vi "Close Network Interface.vi"(8 "error in (no error)":errorcluster, 11 "Network Interface":refnum<data-value>) -> (0 "error out":errorcluster)   [LabVIEW 2017, in "Network Interface.lvlib" / "Network Interface.lvclass"]
uses:
  <vilib>/gpm_packages/@cs/Network-Sink/Source/Network Interface/Network Interface/Network Interface.lvclass
  <vilib>/gpm_packages/@cs/Network-Sink/Source/Network Interface/Network Session Handler/Session Handler Message Names ENUM.ctl
  <vilib>/gpm_packages/@cs/Network-Sink/Source/Network Interface/Network Interface/Network Interface.lvclass/Network Interface.ctl
  <vilib>/gpm_packages/@cs/Network-Sink/Source/Network Interface/Message Queue/Message Queue.lvclass/Message Queue.ctl
  05c7863f-13bf-43fd-8f9a-3362d466c09a.vi
  <vilib>/gpm_packages/@cs/Network-Sink/Source/Network Interface/Message Queue/Protected Enqueue.vi
  <vilib>/gpm_packages/@cs/Network-Sink/Source/Network Interface/Network Session Handler/Network Session Handler.lvclass
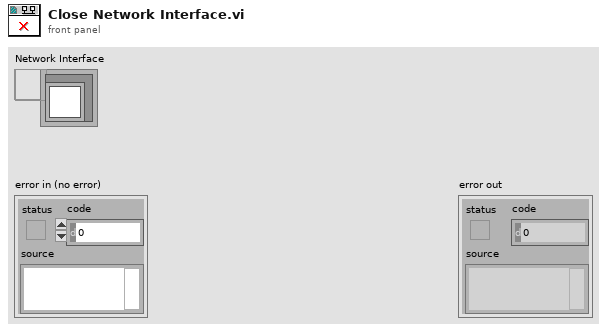
[diagram p1: front panel]
types:
  T1 = typedef "Network Interface.lvlib/Network Session Handler.lvclass/Session Handler Message Names ENUM.ctl" = enum16{"Transmit Message", "Stop", "Handler Shutdown", "Error"}
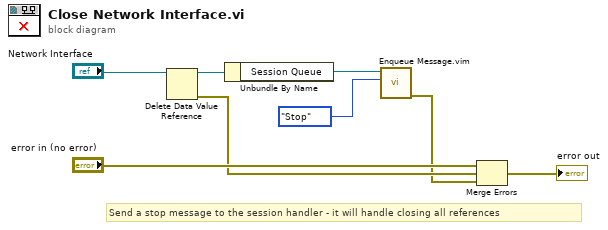
[diagram p0: block diagram]
diagram:
  # "Send a stop message to the session handler - it will handle closing all references"
  n1 = Delete Data Value Reference(data value reference="Network Interface") -> (data value=w6:refnum<class "Network Interface.lvclass">, error out=w5:errorcluster)  [unwired: 1 in]
  n2 = Unbundle By Name(w6) -> ("Session Queue"=w3:refnum<class "Message Queue.lvclass">)
  n3 = call "Enqueue Message.vim"("Msg"=Session_Handler_Message_Names_ENUM."Stop" ("Session Handler Messages"), "Message Queue in"=w3) -> ("error out"=w2:errorcluster)  [unwired: 8 in, 1 out]
  n4 = Merge Errors("error in (no error)", w5, w2) -> (→"error out":errorcluster)
